vi "数据查询.vi"() -> ()   [LabVIEW 2016, in "数据查询.lvlib"]
uses:
  <vilib>/Utility/sysdir.llb/System Directory Type.ctl
  <vilib>/Utility/miscctls.llb/LVPointTypeDef.ctl
  var/holding var.vi
  <vilib>/ptbypt/NI_PtbyPt.lvlib
panel:
  out "布尔":bool
  in  "设置按钮":bool
  in  "标识说明":bool
  in  "数据查询菜单":enum32{"数据查询", "仪器数据", "仪器日志", "报警信息", "校准日志"}(xcontrol)
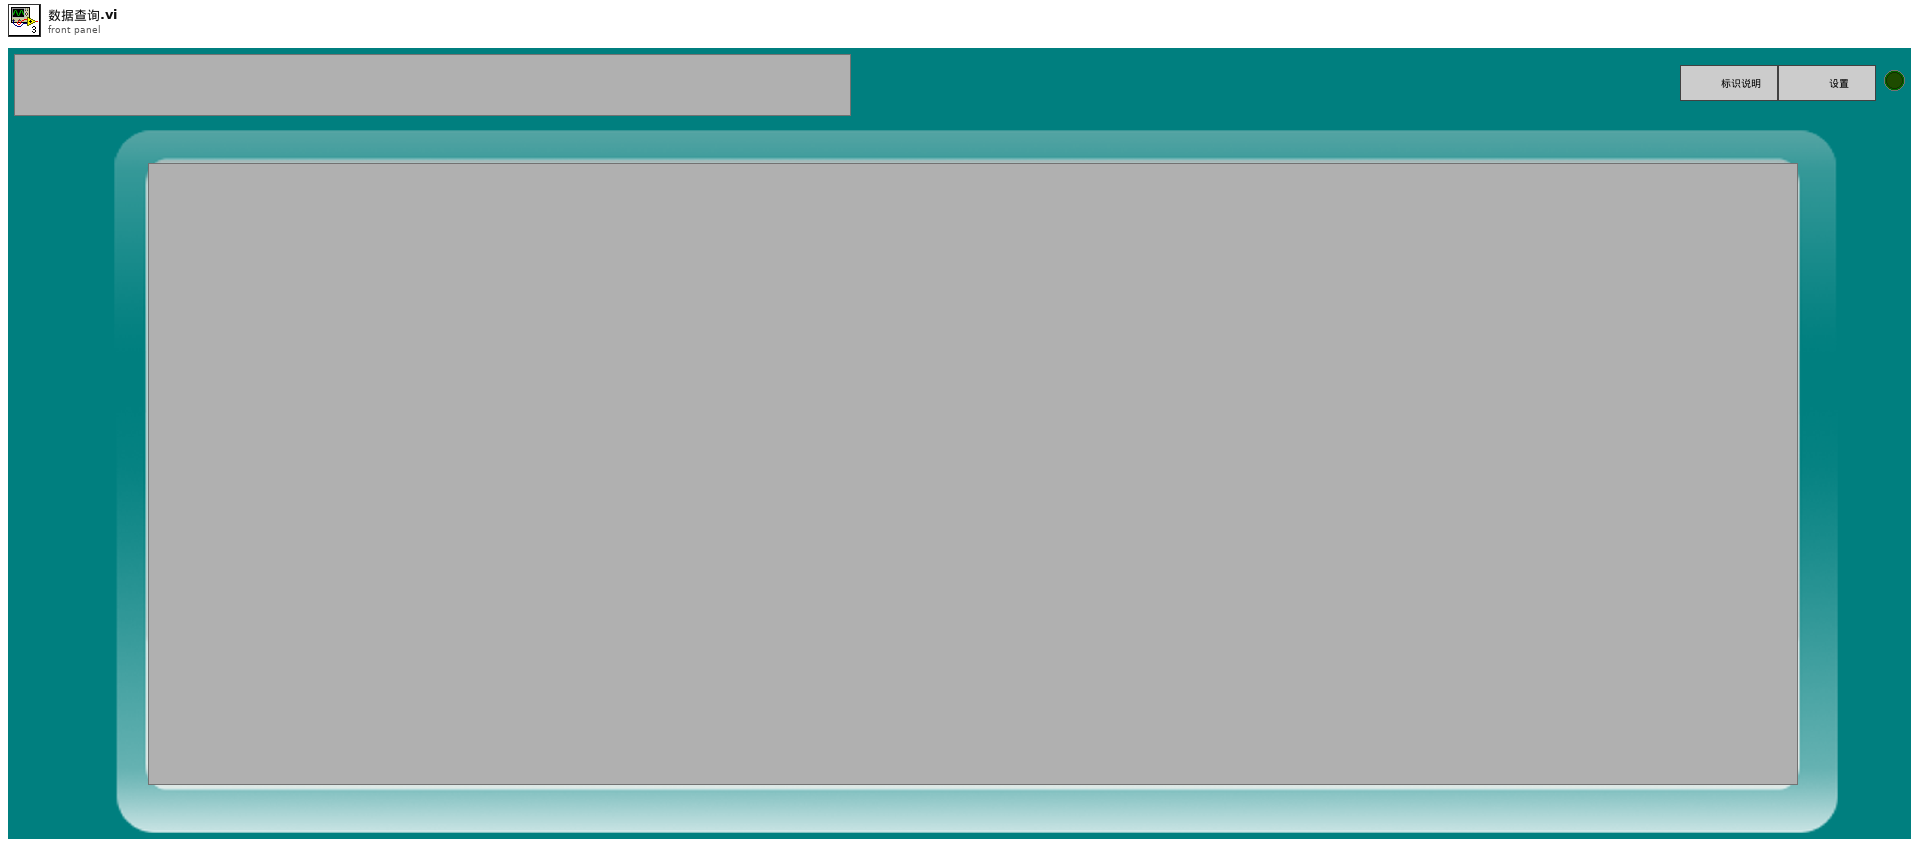
[diagram p1: front panel]
types:
  T1 = typedef "LVPointTypeDef.ctl" = cluster{"Horizontal":i16, "Vertical":i16}
  T2 = typedef "LVDateTimeRec.ctl" = cluster{"秒数的小数部分":dbl, "秒":i32, "分":i32, "时":i32, "日":i32, "月":i32, "年":i32, "天数（周）":i32, "天数（年）":i32, "DST":i32}
  T3 = typedef "System Directory Type.ctl" = i32
  T4 = enum32{"Bad", "Idle", "Run top level", "Running"}
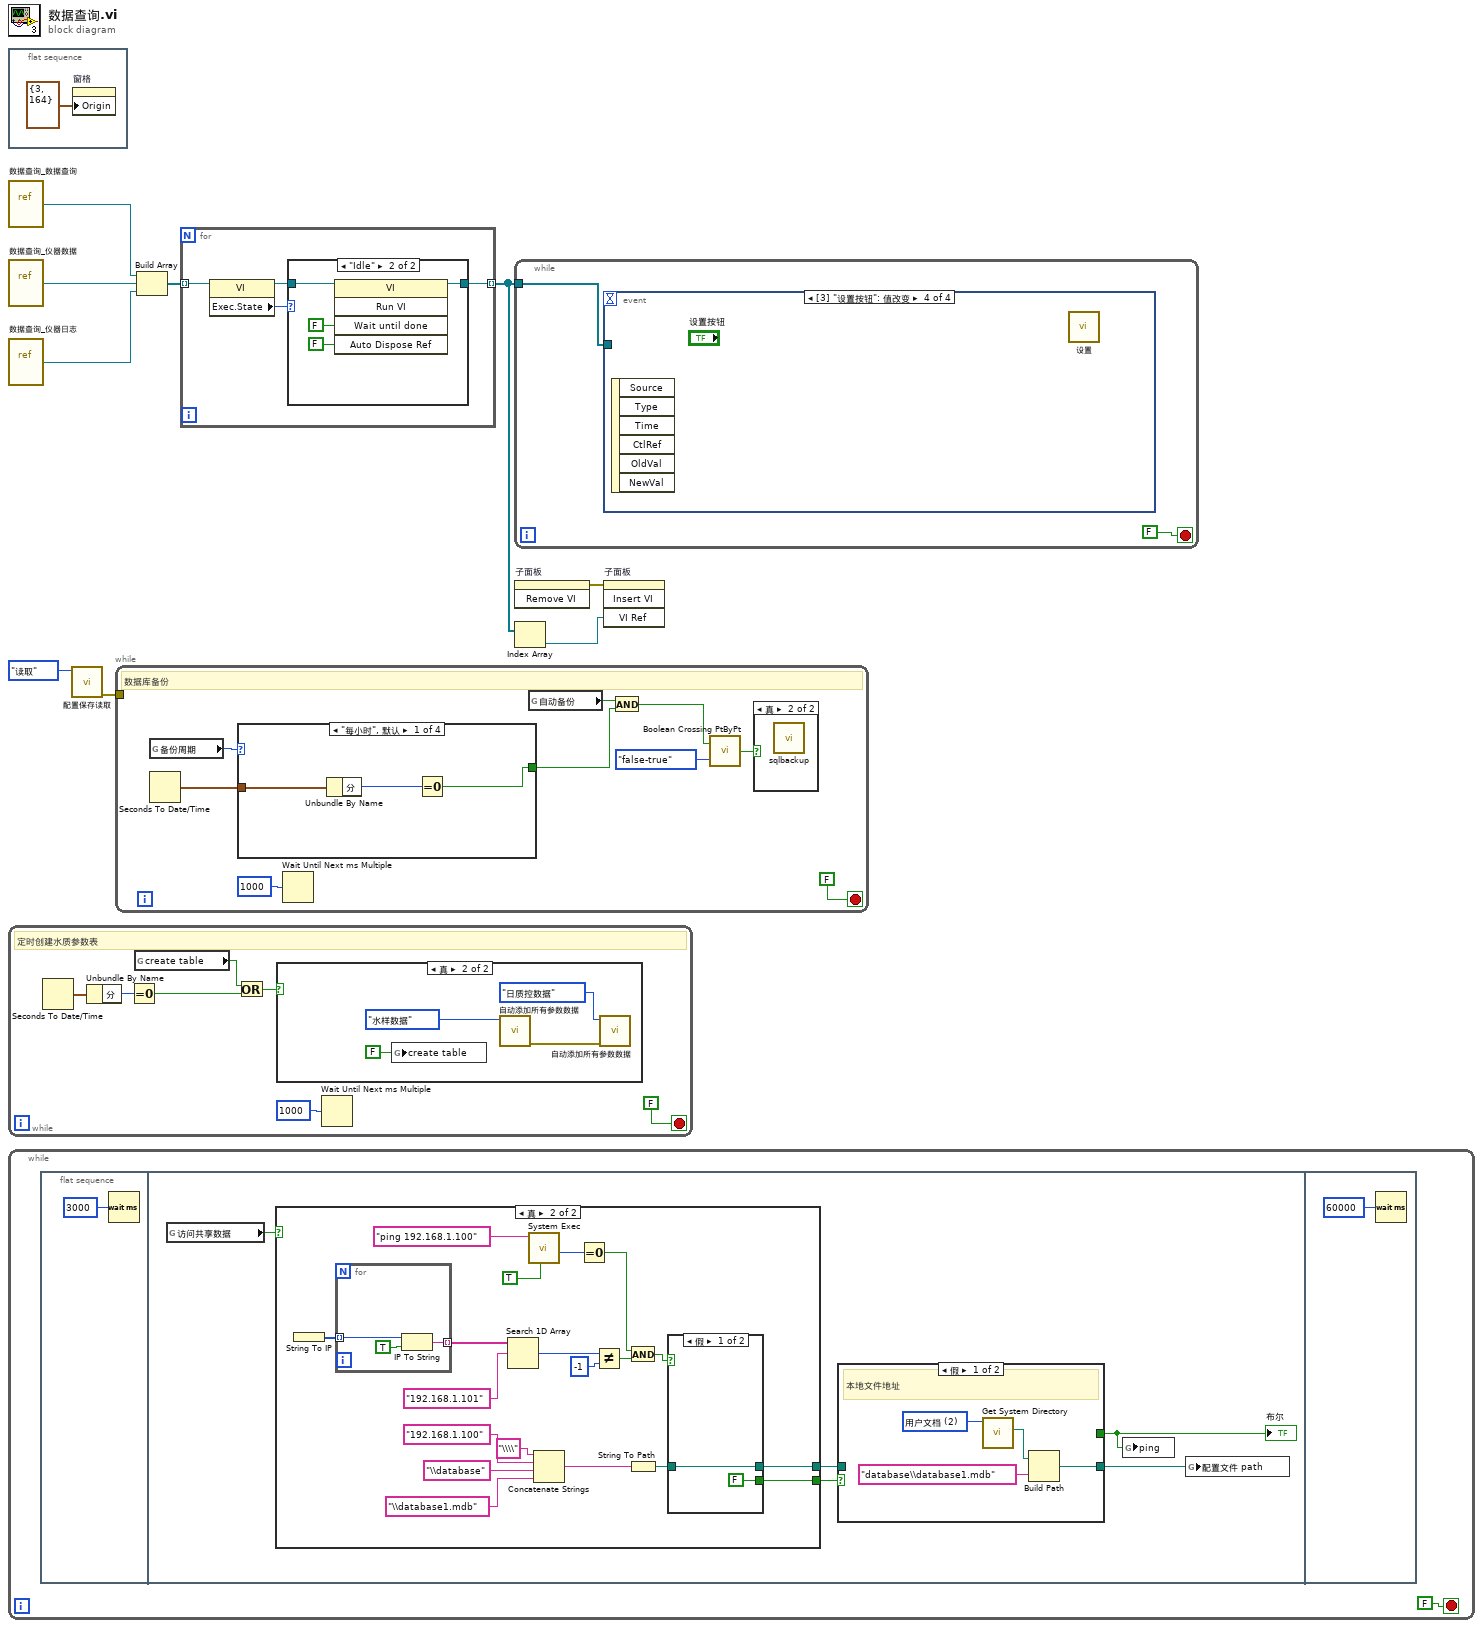
[diagram p0: block diagram]
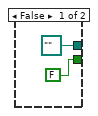
[diagram p2: hidden frame]
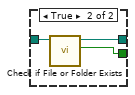
[diagram p3: hidden frame]
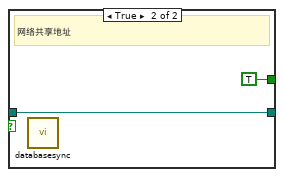
[diagram p4: hidden frame]
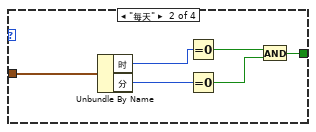
[diagram p6: hidden frame]
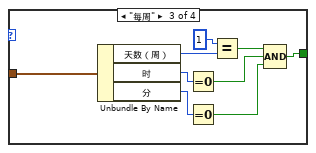
[diagram p7: hidden frame]
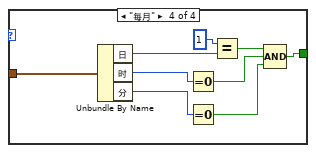
[diagram p8: hidden frame]
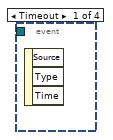
[diagram p11: hidden frame]
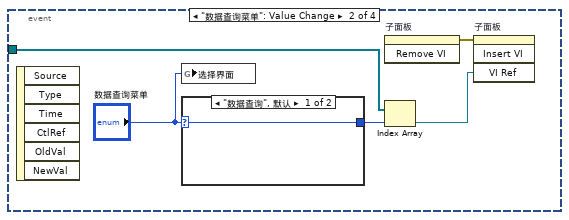
[diagram p12: hidden frame]
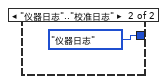
[diagram p13: hidden frame]
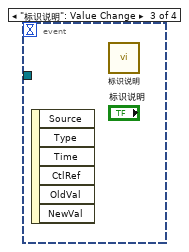
[diagram p14: hidden frame]
diagram:
  n1 = flat-sequence {
    frame #0 {
      n2 = property on="窗格" class="Pane"("Origin"=T1 {"Horizontal"=3, "Vertical"=164} ("原点")) -> ()  [unwired: 2 in, 2 out]
    }
  }
  n3 = vi-ref "数据查询_数据查询.vi"() -> (w6:refnum<vi>)
  n4 = vi-ref "数据查询_仪器数据.vi"() -> (w4:refnum<vi>)
  n5 = vi-ref "数据查询_仪器日志.vi"() -> (w3:refnum<vi>)
  n6 = while {
    stop <- FALSE stop-if-true
    # "定时创建水质参数表"
    n7 = Seconds To Date/Time() -> (date time rec=w17:T2)  [unwired: 2 in]
    n8 = Unbundle By Name(w17) -> ("分"=w16:i32)
    n9 = Equal To 0?(x=w16) -> (x = 0?=w13:bool)
    n10 = global read "全局变量.vi" "create table"() -> (w12:bool)
    n11 = Or(x=w12, y=w13) -> (x .or. y?=w14:bool)
    n12 = case shown="真" w14 {
      frame False {
      }
      frame True {
        n13 = global write "全局变量.vi" "create table"(FALSE ("create table")) -> ()
        n14 = call "自动添加所有参数数据.vi"("数据类别"=enum16{"水样数据", "日质控数据"}."水样数据") -> ("错误输出"=w21:errorcluster)  [unwired: 10 in]
        n15 = call "自动添加所有参数数据.vi"("error in (no error)"=w21, "数据类别"=enum16{"水样数据", "日质控数据"}."日质控数据") -> ()  [unwired: 9 in, 1 out]
      }
    }
    n16 = Wait Until Next ms Multiple(millisecond multiple=u32 1000 ("毫秒倍数")) -> ()  [unwired: 1 out]
  }
  n17 = while {
    stop <- FALSE stop-if-true
    n18 = flat-sequence {
      frame #0 {
        n19 = Wait (ms)(milliseconds to wait=u32 3000 ("等待时间（毫秒）")) -> ()  [unwired: 1 out]
      }
      frame #1 {
        n20 = global read "全局变量.vi" "访问共享数据"() -> (w25:bool)
        n21 = case shown="真" w25 {
          tunnel: [path "" ("dup path") w43] -> w28
          tunnel: [FALSE ("file or folder exists?") w42] -> w27
          frame False {
          }
          frame True {
            n22 = String To IP() -> (0:w36:u32[])  [unwired: 1 in]
            n23 = for {
              tunnel: w36 -> [w52] mode=indexing
              tunnel: [w51] -> w35 mode=indexing
              n24 = IP To String(1:TRUE ("句点符号？(F)"), 2:w52) -> (0:w51:string)
            }
            n25 = Search 1D Array(1D array=w35, element="192.168.1.101" ("command line")) -> (index of element=w33:i32)  [unwired: 1 in]
            n26 = call <vilib>:"System Exec.vi"("run minimized? (F)"=TRUE, "command line"="ping 192.168.1.100") -> ("return code"=w39:i32)  [unwired: 6 in, 3 out]
            n27 = Concatenate Strings("\\\\" ("字符串"), "192.168.1.100" ("名称"), "\\database" ("字符串"), "\\database1.mdb" ("名称或相对路径")) -> (w48:string)
            n28 = Equal To 0?(x=w39) -> (x = 0?=w38:bool)
            n29 = Not Equal?(x=w33, y=-1) -> (x != y?=w31:bool)
            n30 = And(x=w38, y=w31) -> (x .and. y?=w37:bool)
            n31 = String To Path(string=w48) -> (path=w45:path)
            n32 = case shown="假" w37 {
              tunnel: w45 -> [w53 w57]
              tunnel: [w53 w56] -> w43
              tunnel: [FALSE w55] -> w42
              frame False {
              }
              frame True {
                n33 = call <vilib>:"Check if File or Folder Exists.vi"("path"=w57) -> ("file or folder exists?"=w55:bool, "dup path"=w56:path)  [unwired: 8 in, 1 out]
              }
            }
          }
        }
        n34 = case shown="假" w27 {
          tunnel: w28 -> [_ w63]
          tunnel: [w60 w63] -> w26
          tunnel: [_ TRUE] -> w24
          frame False {
            w58 = T3 2 items=["用户目录"=0, "用户桌面"=1, "用户文档"=2, "用户应用程序数据"=3, "用户设置"=4, "用户临时目录"=5, "公共文档"=6, "公共应用程序数据"=7, "公共设置"=8, "公共缓存"=13, "系统核心库"=9, "系统安装库"=10, "应用程序文件"=11, "启动盘根目录"=12] ("system directory type")
            # "本地文件地址"
            n35 = call <vilib>:"Get System Directory.vi"("system directory type"=w58) -> ("system directory"=w59:path)  [unwired: 10 in]
            n36 = Build Path(base path=w59, name or relative path="database\\database1.mdb" ("名称或相对路径")) -> (appended path=w60:path)
          }
          frame True {
            # "网络共享地址"
            n37 = call "databasesync.vi"() -> ()  [unwired: 12 in]
          }
        }
        "布尔" <- w24
        n38 = global write "全局变量.vi" "ping"(w24) -> ()
        n39 = global write "全局变量.vi" "配置文件 path"(w26) -> ()
      }
      frame #2 {
        n40 = Wait (ms)(milliseconds to wait=u32 60000 ("等待时间（毫秒）")) -> ()  [unwired: 1 out]
      }
    }
  }
  n41 = call "配置保存读取.vi"("配置"=enum16{"读取", "写入"}."读取") -> ("error out"=w1:errorcluster)  [unwired: 10 in]
  n42 = while {
    tunnel: w1 -> [_]
    stop <- FALSE stop-if-true
    # "数据库备份"
    n43 = global read "holding var.vi" "备份周期"() -> (w72:enum16{"每小时", "每天", "每周", "每月"})
    n44 = Seconds To Date/Time() -> (date time rec=w67:T2)  [unwired: 2 in]
    n45 = case shown="\"每小时\", 默认" w72 {
      tunnel: w67 -> [w76 w82 w91 w100]
      tunnel: [w74 w77 w83 w92] -> w66
      frame "每小时", Default {
        n46 = Unbundle By Name(w76) -> ("分"=w75:i32)
        n47 = Equal To 0?(x=w75) -> (x = 0?=w74:bool)
      }
      frame "每天" {
        n48 = Unbundle By Name(w82) -> ("时"=w80:i32, "分"=w81:i32)
        n49 = Equal To 0?(x=w80) -> (x = 0?=w78:bool)
        n50 = Equal To 0?(x=w81) -> (x = 0?=w79:bool)
        n51 = And(x=w78, y=w79) -> (x .and. y?=w77:bool)
      }
      frame "每周" {
        n52 = Unbundle By Name(w91) -> ("天数（周）"=w90:i32, "时"=w88:i32, "分"=w87:i32)
        n53 = Equal To 0?(x=w88) -> (x = 0?=w85:bool)
        n54 = Equal To 0?(x=w87) -> (x = 0?=w84:bool)
        n55 = Equal?(x=1, y=w90) -> (x = y?=w86:bool)
        n56 = Compound Arithmetic op=AND ("复合运算")(w86, w85, w84) -> (w83:bool)
      }
      frame "每月" {
        n57 = Unbundle By Name(w100) -> ("日"=w99:i32, "时"=w97:i32, "分"=w96:i32)
        n58 = Equal To 0?(x=w97) -> (x = 0?=w94:bool)
        n59 = Equal To 0?(x=w96) -> (x = 0?=w93:bool)
        n60 = Equal?(x=1, y=w99) -> (x = y?=w95:bool)
        n61 = Compound Arithmetic op=AND ("复合运算")(w95, w94, w93) -> (w92:bool)
      }
    }
    n62 = Wait Until Next ms Multiple(millisecond multiple=u32 1000 ("毫秒倍数")) -> ()  [unwired: 1 out]
    n63 = global read "holding var.vi" "自动备份"() -> (w71:bool)
    n64 = And(x=w71, y=w66) -> (x .and. y?=w70:bool)
    n65 = call <vilib>:"Boolean Crossing PtByPt.vi"("direction"=enum16{"either", "false-true", "true-false"}."false-true", "input"=w70) -> ("crossing"=w68:bool)  [unwired: 1 in]
    n66 = case shown="真" w68 {
      frame False {
      }
      frame True {
        n67 = call "sqlbackup.vi"() -> ()  [unwired: 11 in, 1 out]
      }
    }
  }
  n68 = Build Array(w6, w4, w3) -> (w5:refnum<vi>[])
  n69 = for {
    tunnel: w5 -> [w104] mode=indexing
    tunnel: [w101] -> w8 mode=indexing
    n70 = property class="VI"(reference=w104) -> (reference out=w102:refnum<vi>, "Exec.State"=w103:T4)  [unwired: 1 in, 1 out]
    n71 = case shown="\"Idle\"" w103 {
      tunnel: w102 -> [w105 w107]
      tunnel: [w105 w106] -> w101
      frame "Bad", Default {
      }
      frame "Idle" {
        n72 = invoke class="VI" method="Run VI"(reference=w107, "Wait until done"=FALSE ("结束前等待"), "Auto Dispose Ref"=FALSE ("自动销毁引用")) -> (reference out=w106:refnum<vi>)  [unwired: 2 in, 4 out]
      }
    }
  }
  n73 = while {
    tunnel: w8 -> [w110]
    stop <- FALSE stop-if-true
    n74 = event shown="[3] \"设置按钮\": 值改变" {
      selector: _ -> [_ _ _ _]
      dyn-events: _ -> [_ _ _ _]
      timeout: _ -> [_ _ _ _]
      tunnel: w110 -> [_ w116 _ _]
      event Timeout {
        n75 = event-data() -> ()  [unwired: 1 in, 3 out]
      }
      event "数据查询菜单": Value Change {
        n76 = event-data() -> ()  [unwired: 1 in, 6 out]
        n77 = global write "全局变量.vi" "选择界面"("数据查询菜单") -> ()
        n78 = case shown="\"数据查询\", 默认" "数据查询菜单" {
          selector: "数据查询菜单" -> [w117 _]
          tunnel: [w117 enum32{"数据查询", "仪器数据", "仪器日志", "报警信息", "校准日志"}."仪器日志" ("数据查询菜单")] -> w113
          frame "数据查询", Default {
          }
          frame "仪器日志".."校准日志" {
          }
        }
        n79 = invoke on="子面板" class="SubPnl" method="Remove VI"() -> (error out=w114:errorcluster)  [unwired: 3 in, 2 out]
        n80 = Index Array(array=w116, index=w113) -> (element=w115:refnum<vi>)
        n81 = invoke on="子面板" class="SubPnl" method="Insert VI"(error in=w114, "VI Ref"=w115) -> ()  [unwired: 2 in, 4 out]
      }
      event "标识说明": Value Change {
        n82 = event-data() -> ()  [unwired: 1 in, 6 out]
        n83 = call "标识说明.vi"() -> ()  [unwired: 12 in]
      }
      event "设置按钮": Value Change {
        n84 = event-data() -> ()  [unwired: 1 in, 6 out]
        n85 = call "设置.vi"() -> ()  [unwired: 12 in]
      }
    }
  }
  n86 = invoke on="子面板" class="SubPnl" method="Remove VI"() -> (error out=w9:errorcluster)  [unwired: 3 in, 2 out]
  n87 = Index Array(array=w8) -> (element=w7:refnum<vi>)  [unwired: 1 in]
  n88 = invoke on="子面板" class="SubPnl" method="Insert VI"(error in=w9, "VI Ref"=w7) -> ()  [unwired: 2 in, 4 out]
